vi "DrivePID.vi"(0 "Ldrive Encoder":dbl, 2 "Max Speed":dbl=0.5, 5 "Rdrive Encoder":dbl, 7 "Compensate":bool, 9 "SetpointLeft":dbl format="%.2f", 11 "SetpointRight":dbl format="%.2f") -> (6 "Left Out":dbl, 8 "Right Out":dbl, 15 "Done":bool)   [LabVIEW 2015]
uses:
  <vilib>/addons/control/pid/pid.llb/PID (DBL).vi
  <vilib>/addons/control/pid/NI_PID_pid.lvlib
panel:
  in  "RightDriveRefNum":string="My Encoder RefNum"
  in  "LeftDriveRefNum":string="My Encoder RefNum"
  in  "PID gains for motor gain":T1={"proportional gain (Kc)"=1.0, "integral time (Ti, min)"=0.01, "derivative time (Td, min)"=0.0} {"derivative time (Td, min)" format="%.3f"; "integral time (Ti, min)" format="%.3f"; "proportional gain (Kc)" format="%.3f"}
  in  "PID gains Right":T1={"proportional gain (Kc)"=0.5, "integral time (Ti, min)"=0.0325, "derivative time (Td, min)"=0.001} {"derivative time (Td, min)" format="%.3f"; "integral time (Ti, min)" format="%.7f"; "proportional gain (Kc)" format="%.3f"}
  out "Right Chart":dbl(graph)
  out "Left Chart":dbl(graph)
  in  "PID gains Left":T1={"proportional gain (Kc)"=0.5, "integral time (Ti, min)"=0.0325, "derivative time (Td, min)"=0.001} {"derivative time (Td, min)" format="%.3f"; "integral time (Ti, min)" format="%.7f"; "proportional gain (Kc)" format="%.3f"}
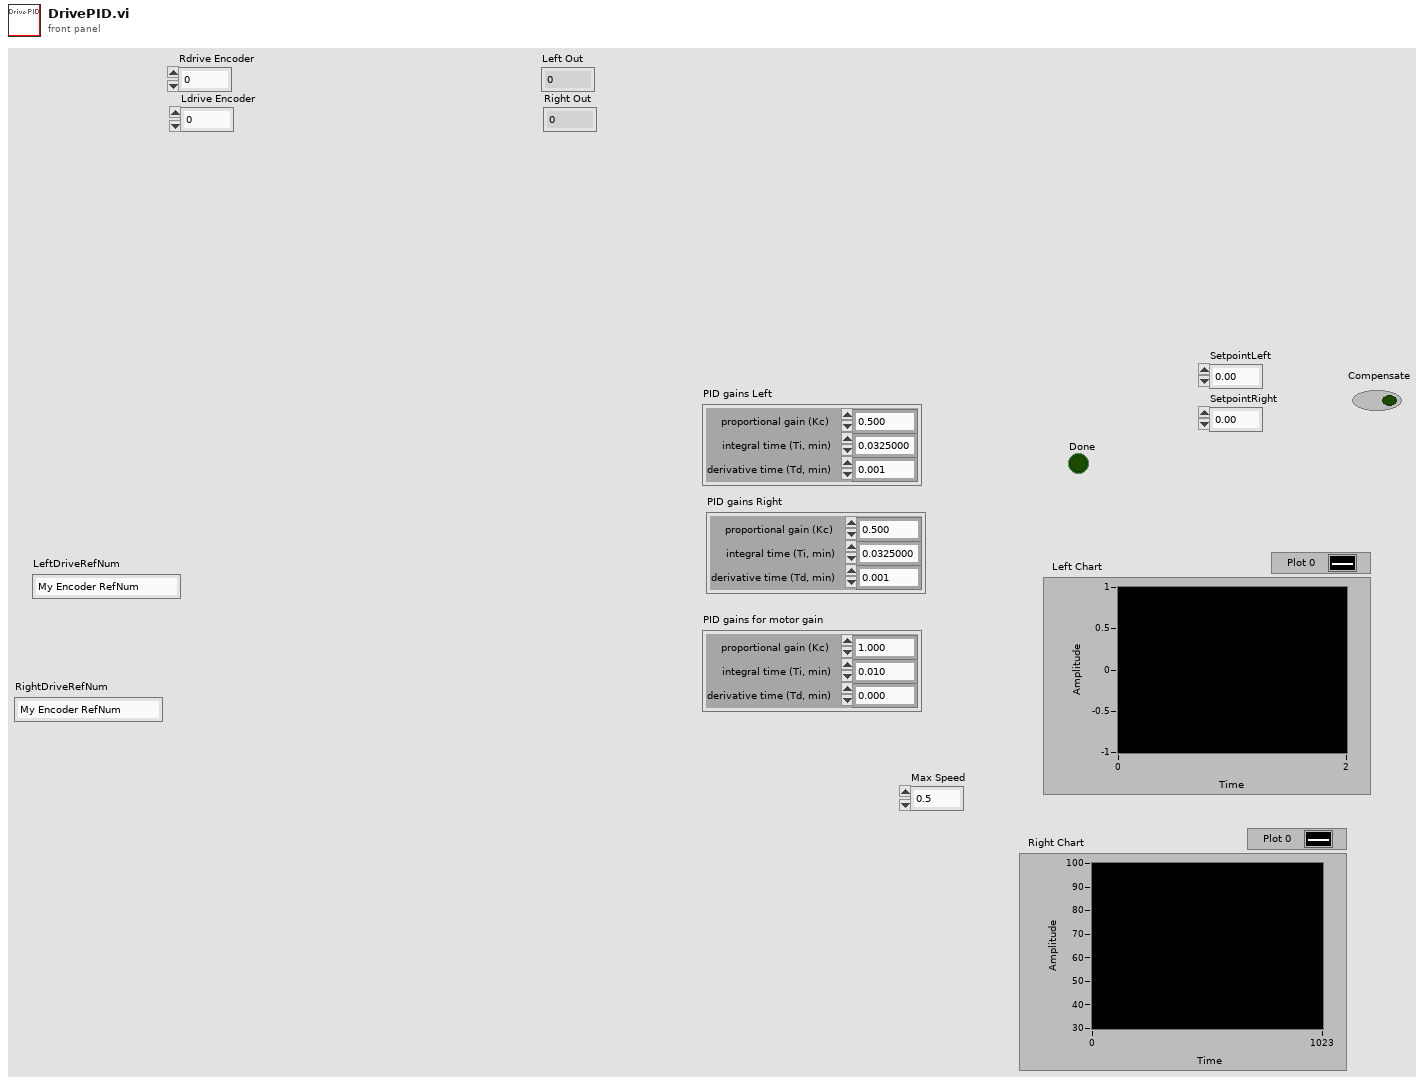
[diagram p1: front panel]
types:
  T1 = cluster{"proportional gain (Kc)":dbl, "integral time (Ti, min)":dbl, "derivative time (Td, min)":dbl}
  T2 = typedef "WPI_EncoderDevRef.ctl" = cluster{"DevStatus":errorcluster, "EncoderIndex":T3, "CounterIndex":T4, "DistancePerCount":dbl, "Decoding Type":T5}
  T3 = typedef "FPGA_EncoderIdx.ctl" = enum8{"Enc 0", "Enc 1", "Enc 2", "Enc 3", "Enc 4", "Enc 5", "Enc 6", "Enc 7", "Invalid"}
  T4 = typedef "FPGA_CounterCtrSystemIndex.ctl" = enum8{"Ctr 0", "Ctr 1", "Ctr 2", "Ctr 3", "Ctr 4", "Ctr 5", "Ctr 6", "Ctr 7", "Invalid"}
  T5 = typedef "WPI_EncoderType.ctl" = enum16{"1x", "2x", "4x"}
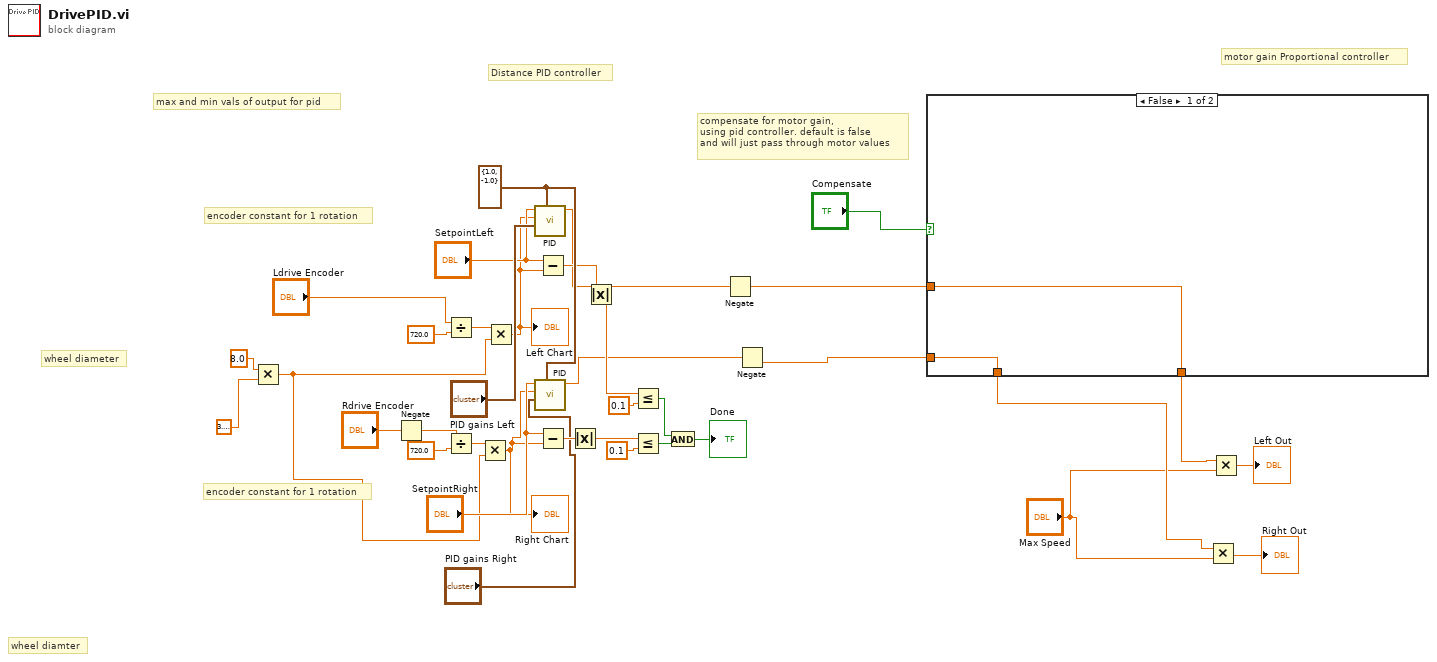
[diagram p0: block diagram]
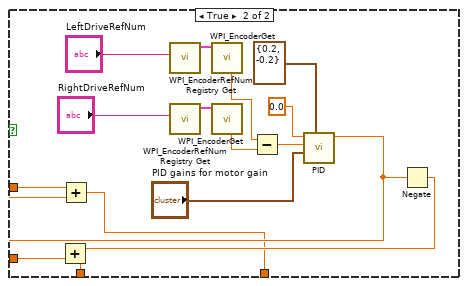
[diagram p2: hidden frame]
diagram:
  w34 = cluster{"output high":dbl, "output low":dbl} {"output high"=1.0, "output low"=-1.0} ("output range")
  # "compensate for motor gain,\nusing pid controller. default is false\nand will just pass through motor values"
  # "max and min vals of output for pid"
  # "encoder constant for 1 rotation"
  # "encoder constant for 1 rotation"
  # "wheel diamter"
  # "wheel diameter"
  # "motor gain Proportional controller"
  # "Distance PID controller"
  n1 = Multiply(x=8.0, y=3.141592653589793) -> (x*y=w6:dbl)
  n2 = Negate(x="Rdrive Encoder") -> (-x=w3:dbl)
  n3 = Divide(x="Ldrive Encoder", y=720.0) -> (x/y=w20:dbl)
  n4 = Divide(x=w3, y=720.0) -> (x/y=w18:dbl)
  n5 = Multiply(x=w18, y=w6) -> (x*y=w16:dbl)
  "Right Chart" <- w16
  n6 = Multiply(x=w20, y=w6) -> (x*y=w19:dbl)
  "Left Chart" <- w19
  n7 = call-poly <vilib>:"PID.vi"("output range"=w34, "PID gains"="PID gains Left", "process variable"=w19, "setpoint"="SetpointLeft") -> ("output"=w15:dbl)  [unwired: 6 in, 1 out]
  n8 = call-poly <vilib>:"PID.vi"("output range"=w34, "PID gains"="PID gains Right", "process variable"=w16, "setpoint"="SetpointRight") -> ("output"=w4:dbl)  [unwired: 6 in, 1 out]
  n9 = Subtract(x="SetpointLeft", y=w19) -> (x-y=w32:dbl)
  n10 = Subtract(x="SetpointRight", y=w16) -> (x-y=w27:dbl)
  n11 = Absolute Value(x=w27) -> (abs(x)=w21:dbl)
  n12 = Absolute Value(x=w32) -> (abs(x)=w22:dbl)
  n13 = Less Or Equal?(x=w22, y=0.1) -> (x <= y?=w29:bool)
  n14 = Less Or Equal?(x=w21, y=0.1) -> (x <= y?=w30:bool)
  n15 = And(x=w29, y=w30) -> (x .and. y?=→"Done":bool)
  n16 = Negate(x=w15) -> (-x=w7:dbl)
  n17 = Negate(x=w4) -> (-x=w2:dbl)
  n18 = case shown="False" "Compensate" {
    tunnel: w2 -> [w37 w44]
    tunnel: [w37 w42] -> w12
    tunnel: w7 -> [w38 w41]
    tunnel: [w38 w39] -> w13
    frame False {
    }
    frame True {
      n19 = call <vilib>:"WPI_EncoderRefNum Registry Get.vi"("refnum name"="LeftDriveRefNum") -> ("EncoderDevRef"=w53:T2)  [unwired: 9 in, 1 out]
      n20 = call <vilib>:"WPI_EncoderRefNum Registry Get.vi"("refnum name"="RightDriveRefNum") -> ("EncoderDevRef"=w50:T2)  [unwired: 9 in, 1 out]
      n21 = call <vilib>:"WPI_EncoderGet.vi"("EncoderDevRef"=w53) -> ("Rate"=w48:dbl)  [unwired: 5 in, 5 out]
      n22 = call <vilib>:"WPI_EncoderGet.vi"("EncoderDevRef"=w50) -> ("Rate"=w47:dbl)  [unwired: 5 in, 5 out]
      n23 = Subtract(x=w48, y=w47) -> (x-y=w45:dbl)
      n24 = call-poly <vilib>:"PID.vi"("output range"=cluster{"output high":dbl, "output low":dbl} {"output high"=0.2, "output low"=-0.2}, "PID gains"="PID gains for motor gain", "process variable"=w45, "setpoint"=0.0) -> ("output"=w40:dbl)  [unwired: 6 in, 1 out]
      n25 = Add(x=w41, y=w40) -> (x+y=w39:dbl)
      n26 = Negate(x=w40) -> (-x=w43:dbl)
      n27 = Add(x=w43, y=w44) -> (x+y=w42:dbl)
    }
  }
  n28 = Multiply(x=w12, y="Max Speed") -> (x*y=→"Right Out":dbl)
  n29 = Multiply(x=w13, y="Max Speed") -> (x*y=→"Left Out":dbl)
